vi "Set Value.vi"(8 "error in (no error)":errorcluster, 9 "Value":variant, 10 "Name":string, 11 "Data Reference":T1) -> (0 "error out":errorcluster)   [LabVIEW 2016, in "System.lvlib"]
uses:
  System.lvlib
  Controls/Control_Variant Data Reference.ctl
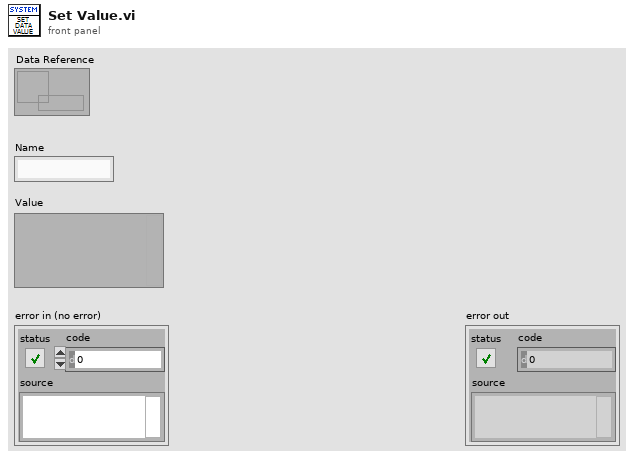
[diagram p1: front panel]
types:
  T1 = typedef "System.lvlib/Control_Variant Data Reference.ctl" = refnum<data-value>
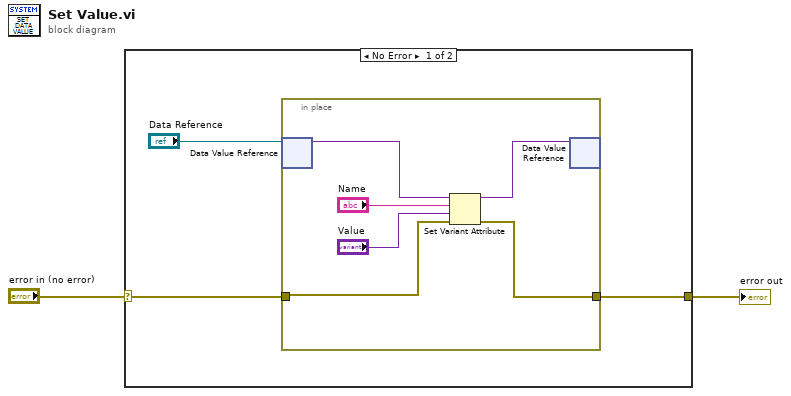
[diagram p0: block diagram]
diagram:
  n1 = case shown="No Error" "error in (no error)" {
    selector: "error in (no error)" -> [w4 w12]
    tunnel: [w3 w12] -> w1
    frame No Error {
      n2 = in-place {
        in-place-border: w4 -> [w7]
        in-place-border: [w6] -> w3
        n3 = in-place-dvr #1("Data Reference") -> (w11:variant)  [unwired: 1 out]
        n4 = Set Variant Attribute(Variant=w11, name="Name", value="Value", error in=w7) -> (Variant out=w10:variant, error out=w6:errorcluster)  [unwired: 1 out]
        n5 = in-place-dvr #1(w10) -> ()  [unwired: 2 out]
      }
    }
    frame Error {
    }
  }
  "error out" <- w1
